vi "Loops deaktivieren.vi"(8 "Istwert Controls[]":refnum<vi>[](array[refnum]), 9 "Grenzwert Controls[]":refnum<vi>[](array[refnum]), 10 "Grenzwerte PNS":T1 {"Heizleitung 6:"."Regler" items=["aktiv", "inaktiv"]; "Heizleitung 6:"."Abschalt-Max" format="%#_5g"; "Heizleitung 6:"."Abschalt-Min" format="%#_5g"; "Heizleitung 6:"."Warn-Max" format="%#_5g"; "Heizleitung 6:"."Warn-Min" format="%#_5g"; "Heizleitung 6:"."Sollwert" format="%#_5g"; "Heizleitung 5:"."Regler" items=["aktiv", "inaktiv"]; "Heizleitung 5:"."Abschalt-Max" format="%#_5g"; "Heizleitung 5:"."Abschalt-Min" format="%#_5g"; "Heizleitung 5:"."Warn-Max" format="%#_5g"; "Heizleitung 5:"."Warn-Min" format="%#_5g"; "Heizleitung 5:"."Sollwert" format="%#_5g"; "Heizleitung 4:"."Regler" items=["aktiv", "inaktiv"]; "Heizleitung 4:"."Abschalt-Max" format="%#_5g"; "Heizleitung 4:"."Abschalt-Min" format="%#_5g"; "Heizleitung 4:"."Warn-Max" format="%#_5g"; "Heizleitung 4:"."Warn-Min" format="%#_5g"; "Heizleitung 4:"."Sollwert" format="%#_5g"; "Heizleitung 3:"."Regler" items=["aktiv", "inaktiv"]; "Heizleitung 3:"."Abschalt-Max" format="%#_5g"; "Heizleitung 3:"."Abschalt-Min" format="%#_5g"; "Heizleitung 3:"."Warn-Max" format="%#_5g"; "Heizleitung 3:"."Warn-Min" format="%#_5g"; "Heizleitung 3:"."Sollwert" format="%#_5g"; "Heizleitung 2:"."Regler" items=["aktiv", "inaktiv"]; "Heizleitung 2:"."Abschalt-Max" format="%#_5g"; "Heizleitung 2:"."Abschalt-Min" format="%#_5g"; "Heizleitung 2:"."Warn-Max" format="%#_5g"; "Heizleitung 2:"."Warn-Min" format="%#_5g"; "Heizleitung 2:"."Sollwert" format="%#_5g"; "Heizleitung 1:"."Regler" items=["aktiv", "inaktiv"]; "Heizleitung 1:"."Abschalt-Max" format="%#_5g"; "Heizleitung 1:"."Abschalt-Min" format="%#_5g"; "Heizleitung 1:"."Warn-Max" format="%#_5g"; "Heizleitung 1:"."Warn-Min" format="%#_5g"; "Heizleitung 1:"."Sollwert" format="%#_5g"; "Ventilplatte:"."Regler" items=["aktiv", "inaktiv"]; "Ventilplatte:"."Abschalt-Max" format="%#_5g"; "Ventilplatte:"."Abschalt-Min" format="%#_5g"; "Ventilplatte:"."Warn-Max" format="%#_5g"; "Ventilplatte:"."Warn-Min" format="%#_5g"; "Ventilplatte:"."Sollwert" format="%#_5g"; "Filter:"."Regler" items=["aktiv", "inaktiv"]; "Filter:"."Abschalt-Max" format="%#_5g"; "Filter:"."Abschalt-Min" format="%#_5g"; "Filter:"."Warn-Max" format="%#_5g"; "Filter:"."Warn-Min" format="%#_5g"; "Filter:"."Sollwert" format="%#_5g"}, 11 "Loopkennung":u16[](array[numeric])) -> ()   [LabVIEW 2020, in "PNS.lvlib"]
uses:
  PNS.lvlib
  ObjektKlassen/Steuerung PNS/Anlegengrenzwerte PNS.ctl
  ObjektKlassen/Steuerung PNS/Anlagengrenzwerte Parameteranzeige.ctl
  Visualisierungs Elemente/Zahlen-Eingabefeld.ctl
  ObjektKlassen/Steuerung PNS/Steuerung PNS.lvclass
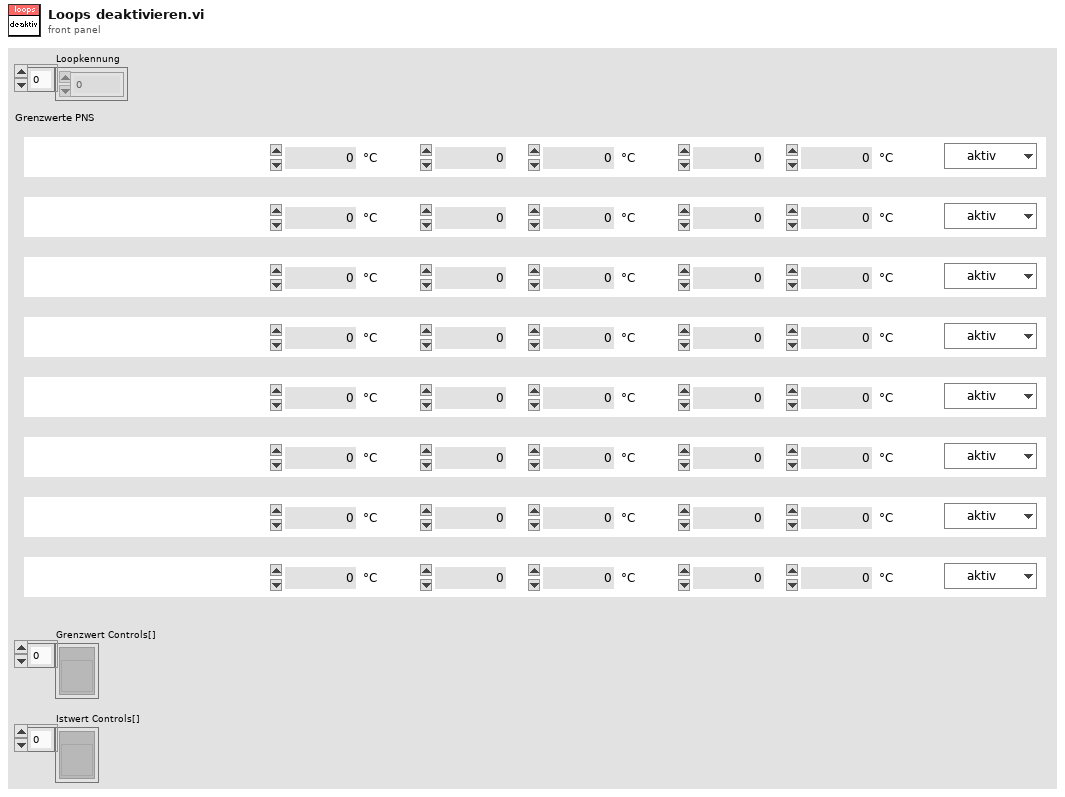
[diagram p1: front panel]
types:
  T1 = typedef "Steuerung PNS.lvclass/Anlegengrenzwerte PNS.ctl" = cluster{"Filter:":T2, "Ventilplatte:":T2, "Heizleitung 1:":T2, "Heizleitung 2:":T2, "Heizleitung 3:":T2, "Heizleitung 4:":T2, "Heizleitung 5:":T2, "Heizleitung 6:":T2}
  T2 = typedef "Steuerung PNS.lvclass/Anlagengrenzwerte Parameteranzeige.ctl" = cluster{"Sollwert":T3, "Warn-Min":T3, "Warn-Max":T3, "Abschalt-Min":T3, "Abschalt-Max":T3, "Regler":u16, "AnlagenParameter":string}
  T3 = typedef "Zahlen-Eingabefeld.ctl" = sgl
  T4 = enum8{"Enabled", "Disabled", "Disabled and Grayed Out"}
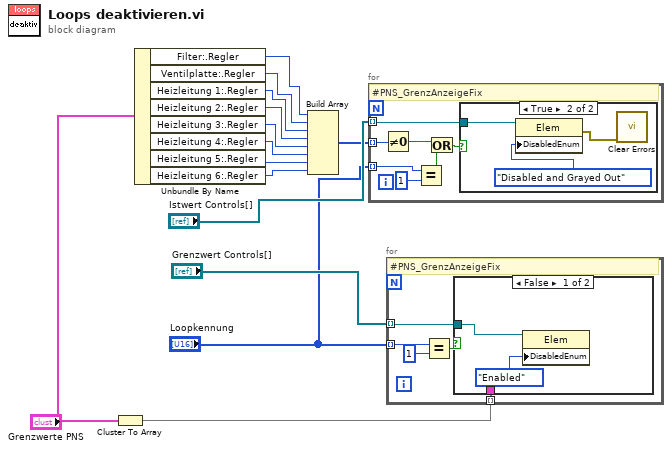
[diagram p0: block diagram]
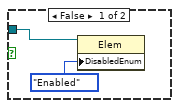
[diagram p2: hidden frame]
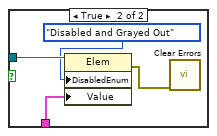
[diagram p3: hidden frame]
diagram:
  n1 = Cluster To Array(cluster="Grenzwerte PNS") -> (array=w1:T2[])
  n2 = Unbundle By Name("Grenzwerte PNS") -> ("Filter:.Regler"=w5:u16, "Ventilplatte:.Regler"=w6:u16, "Heizleitung 1:.Regler"=w7:u16, "Heizleitung 2:.Regler"=w8:u16, "Heizleitung 3:.Regler"=w9:u16, "Heizleitung 4:.Regler"=w10:u16, "Heizleitung 5:.Regler"=w11:u16, "Heizleitung 6:.Regler"=w12:u16)
  n3 = Build Array(w5, w6, w7, w8, w9, w10, w11, w12) -> (w13:u16[])
  n4 = for {
    tunnel: w13 -> [w18] mode=indexing
    tunnel: "Istwert Controls[]" -> [w21] mode=indexing
    tunnel: "Loopkennung" -> [w15] mode=indexing
    # "#PNS_GrenzAnzeigeFix"
    n5 = Not Equal To 0?(x=w18) -> (x != 0?=w17:bool)
    n6 = Equal?(x=w15, y=u16 1) -> (x = y?=w19:bool)
    n7 = Or(x=w17, y=w19) -> (x .or. y?=w16:bool)
    n8 = case shown="True" w16 {
      tunnel: w21 -> [w23 w26]
      frame False {
        n9 = property class="Elem"(reference=w23, "DisabledEnum"=T4."Enabled" ("Deaktiviert")) -> ()  [unwired: 1 in, 2 out]
      }
      frame True {
        n10 = property class="Elem"(reference=w26, "DisabledEnum"=T4."Disabled and Grayed Out" ("Deaktiviert")) -> (error out=w24:errorcluster)  [unwired: 1 in, 1 out]
        n11 = call <vilib>:"Clear Errors.vi"("error in (no error)"=w24) -> ()  [unwired: 5 in, 2 out]
      }
    }
  }
  n12 = for {
    tunnel: "Loopkennung" -> [w31] mode=indexing
    tunnel: "Grenzwert Controls[]" -> [w29] mode=indexing
    tunnel: w1 -> [w27] mode=indexing
    # "#PNS_GrenzAnzeigeFix"
    n13 = Equal?(x=w31, y=u16 1) -> (x = y?=w28:bool)
    n14 = case shown="False" w28 {
      tunnel: w29 -> [w33 w37]
      tunnel: w27 -> [_ w34]
      frame False {
        n15 = property class="Elem"(reference=w33, "DisabledEnum"=T4."Enabled" ("Deaktiviert")) -> ()  [unwired: 1 in, 2 out]
      }
      frame True {
        n16 = property class="Elem"(reference=w37, "DisabledEnum"=T4."Disabled and Grayed Out" ("Deaktiviert"), "Value"=w34) -> (error out=w35:errorcluster)  [unwired: 1 in, 1 out]
        n17 = call <vilib>:"Clear Errors.vi"("error in (no error)"=w35) -> ()  [unwired: 5 in, 2 out]
      }
    }
  }
